vi "need for global func var.vi"() -> ()   [LabVIEW 2013]
uses:
  glopost.vi
panel:
  out "loop sum":dbl
  out "final position":dbl
  in  "stop":bool
  in  "initial position":i32
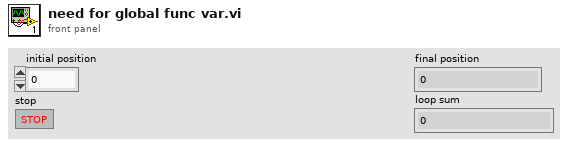
[diagram p1: front panel]
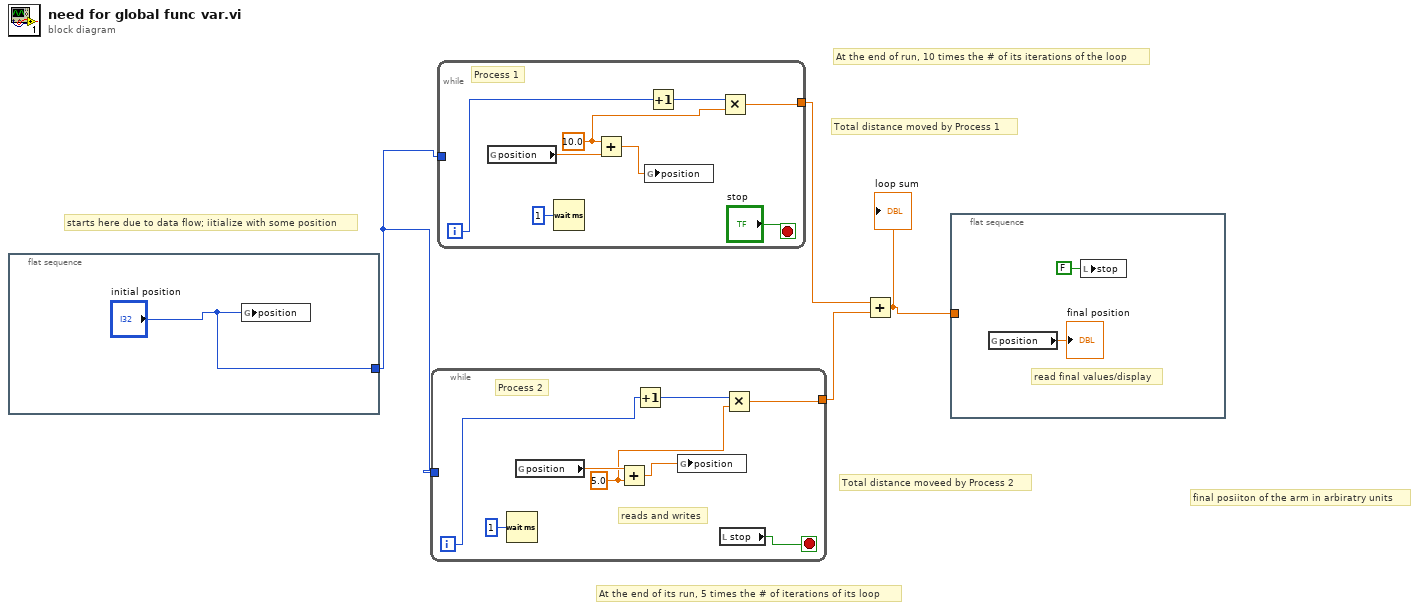
[diagram p0: block diagram]
diagram:
  # "starts here due to data flow; iitialize with some position"
  # "final posiiton of the arm in arbiratry units"
  # "At the end of its run, 5 times the # of iterations of its loop"
  # "At the end of run, 10 times the # of its iterations of the loop"
  # "Total distance moveed by Process 2"
  # "Total distance moved by Process 1"
  n1 = flat-sequence {
    tunnel: ["initial position"] -> w1
    frame #0 {
      n2 = global write "glopost.vi" "position"("initial position") -> ()
    }
  }
  n3 = while {
    tunnel: [w6] -> w3
    tunnel: w1 -> [_]
    i -> [w9]
    stop <- w12 stop-if-true
    w7 = 5.0 ("y")
    # "reads and writes"
    # "Process 2"
    n4 = Wait (ms)(milliseconds to wait=u32 1) -> ()  [unwired: 1 out]
    n5 = global read "glopost.vi" "position"() -> (w11:dbl)
    n6 = Add(x=w11, y=w7) -> (x+y=w10:dbl)
    n7 = Increment(x=w9) -> (x+1=w8:i32)
    n8 = global write "glopost.vi" "position"(w10) -> ()
    n9 = local read "stop"() -> (w12:bool)
    n10 = Multiply(x=w8, y=w7) -> (x*y=w6:dbl)
  }
  n11 = while {
    tunnel: [w14] -> w4
    tunnel: w1 -> [_]
    i -> [w17]
    stop <- "stop" stop-if-true
    w15 = 10.0 ("x")
    # "Process 1"
    n12 = global read "glopost.vi" "position"() -> (w21:dbl)
    n13 = Wait (ms)(milliseconds to wait=u32 1) -> ()  [unwired: 1 out]
    n14 = Add(x=w15, y=w21) -> (x+y=w18:dbl)
    n15 = global write "glopost.vi" "position"(w18) -> ()
    n16 = Increment(x=w17) -> (x+1=w16:i32)
    n17 = Multiply(x=w16, y=w15) -> (x*y=w14:dbl)
  }
  n18 = Add(x=w4, y=w3) -> (x+y=w2:dbl)
  "loop sum" <- w2
  n19 = flat-sequence {
    tunnel: w2 -> [_]
    frame #0 {
      # "read final values/display"
      n20 = global read "glopost.vi" "position"() -> (→"final position":dbl)
      n21 = local write "stop"(FALSE ("stop")) -> ()
    }
  }
